vi "Sort Paths.vi"(9 "Search Expression":string, 10 "filenames":string[](array[string]), 11 "Folder Path":path) -> (2 "File Name":string, 3 "Latest File on Network Folder":path)   [LabVIEW 2012]
doc: "This VI searches the given network folder and finds the latest version."
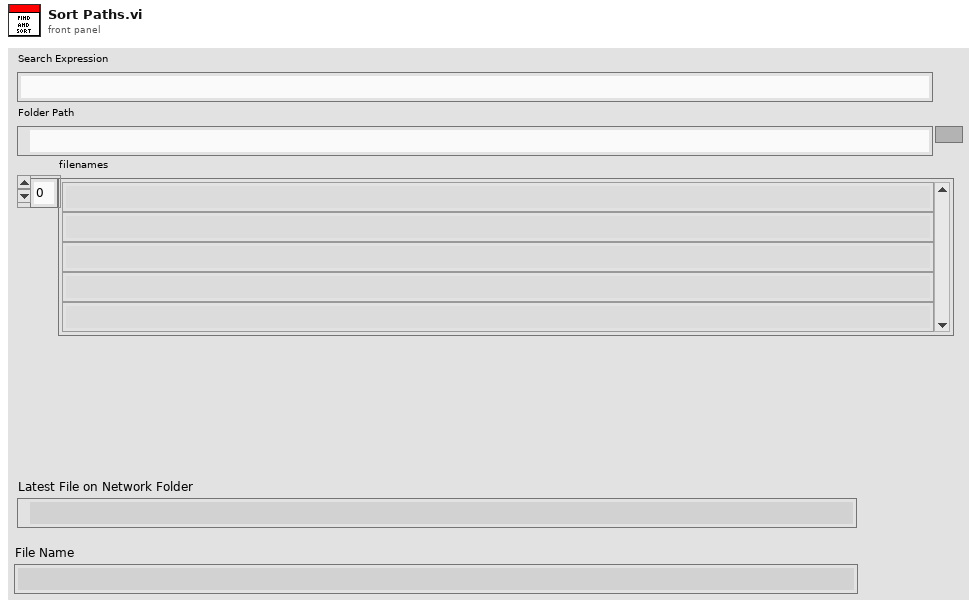
[diagram p1: front panel]
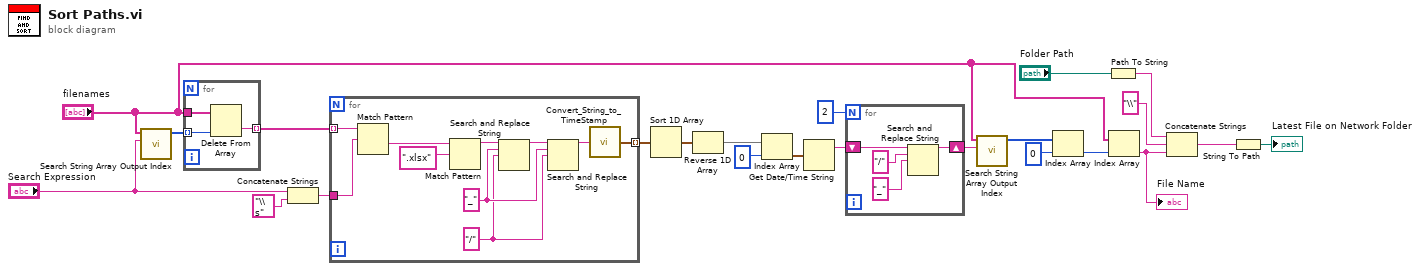
[diagram p0: block diagram]
diagram:
  n1 = call "Search String Array Output Index.vi"("Search Expression"="Search Expression", "filenames"="filenames") -> ("Array"=w19:i32[])  [unwired: 9 in]
  n2 = for {
    tunnel: w19 -> [w26] mode=indexing
    tunnel: "filenames" -> [w25]
    tunnel: [w24] -> w23 mode=indexing
    n3 = Delete From Array(array=w25, index=w26) -> (deleted portion=w24:string)  [unwired: 1 in, 1 out]
  }
  n4 = Concatenate Strings("Search Expression", "\\s" ("string")) -> (w22:string)
  n5 = for {
    tunnel: w23 -> [w36] mode=indexing
    tunnel: w22 -> [w35]
    tunnel: [w28] -> w18 mode=indexing
    w30 = "/" ("replace string (\"\")")
    w31 = "_" ("search string")
    n6 = Match Pattern(string=w36, regular expression=w35) -> (after substring=w33:string)  [unwired: 1 in, 3 out]
    n7 = Match Pattern(string=w33, regular expression=".xlsx") -> (before substring=w32:string)  [unwired: 1 in, 3 out]
    n8 = Search and Replace String(input string=w32, search string=w31, replace string=w30) -> (result string=w29:string)  [unwired: 5 in, 3 out]
    n9 = Search and Replace String(input string=w29, search string=w31, replace string=w30) -> (result string=w27:string)  [unwired: 5 in, 3 out]
    n10 = call "Convert_String_to_TimeStamp.vi"("date/time string"=w27) -> ("Resulting Time Stamp"=w28:timestamp)
  }
  n11 = Sort 1D Array(array=w18) -> (sorted array=w17:timestamp[])
  n12 = Reverse 1D Array(array=w17) -> (reversed array=w16:timestamp[])
  n13 = Index Array(array=w16, index=0) -> (element=w14:timestamp)
  n14 = Get Date/Time String(seconds (now)=w14) -> (date string=w12:string)  [unwired: 2 in, 1 out]
  n15 = for {
    N: 2 -> [_]
    shift-right: [w37] -> w2
    shift-left: w12 -> [w40]
    n16 = Search and Replace String(input string=w40, search string="/" ("replace string (\"\")"), replace string="_" ("search string")) -> (result string=w37:string)  [unwired: 5 in, 3 out]
  }
  n17 = call "Search String Array Output Index.vi"("Search Expression"=w2, "filenames"="filenames") -> ("Array"=w1:i32[])  [unwired: 9 in]
  n18 = Index Array(array=w1, index=0) -> (element=w10:i32)
  n19 = Path To String(path="Folder Path") -> (string=w7:string)
  n20 = Index Array(array="filenames", index=w10) -> (element=w5:string)
  "File Name" <- w5
  n21 = Concatenate Strings(w7, "\\" ("string"), w5) -> (w8:string)
  n22 = String To Path(string=w8) -> (path=→"Latest File on Network Folder":path)
